vi "Update Picked Up Items Display.vi"(8 "error in (no error)":errorcluster, 10 "Item Description":string, 11 "Customer in":refnum<class "Customer.lvclass">) -> (0 "error out":errorcluster, 3 "Customer out":refnum<class "Customer.lvclass">)   [LabVIEW 2023, in "Customer.lvlib" / "Customer.lvclass"]
doc: "Notify Customer's UI handler to update the display of picked up items with <b>Item Description</b>."
uses:
  Customer.lvclass
  Customer.lvclass/Customer.ctl
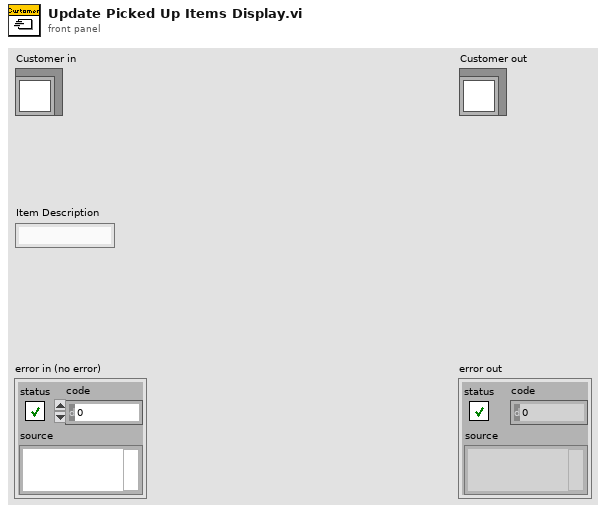
[diagram p1: front panel]
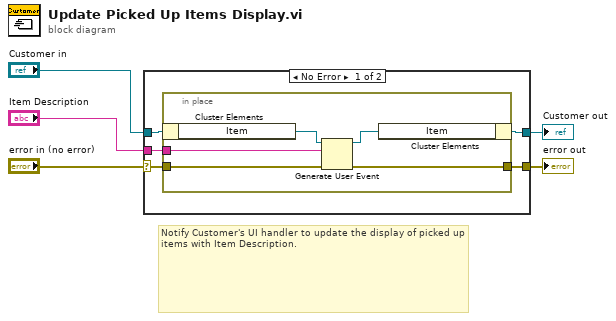
[diagram p0: block diagram]
diagram:
  # "Notify Customer's UI handler to update the display of picked up items with Item Description."
  n1 = case shown="No Error" "error in (no error)" {
    selector: "error in (no error)" -> [w9 w17]
    tunnel: [w8 w17] -> w4
    tunnel: [w6 w16] -> w2
    tunnel: "Customer in" -> [w7 w16]
    tunnel: "Item Description" -> [w10 _]
    frame No Error {
      n2 = in-place "In Place Element Structure" {
        in-place-border: w10 -> [w15]
        in-place-border: w9 -> [w14]
        in-place-border: [w13] -> w8
        n3 = in-place-cluster #1 ("Unbundle / Bundle Elements")(w7) -> ("Item"=w12:refnum<user-event>)
        n4 = Generate User Event(user event=w12, event data cluster=w15, error in=w14) -> (user event out=w11:refnum<user-event>, error out=w13:errorcluster)  [unwired: 1 in]
        n5 = in-place-cluster #1 ("Unbundle / Bundle Elements")("Item"=w11) -> (w6:refnum<class "Customer.lvclass">)
      }
    }
    frame Error {
    }
  }
  "error out" <- w4
  "Customer out" <- w2
